vi "网分校准.vi"(8 "error in (no error)":errorcluster, 11 "network in":refnum<class "network.lvclass">) -> (0 "error out":errorcluster, 3 "network out":refnum<class "network.lvclass">)   [LabVIEW 2015, in "network.lvclass"]
uses:
  network.lvclass
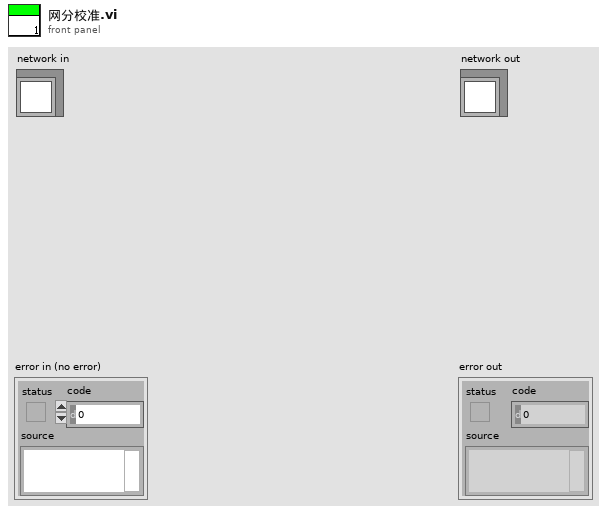
[diagram p1: front panel]
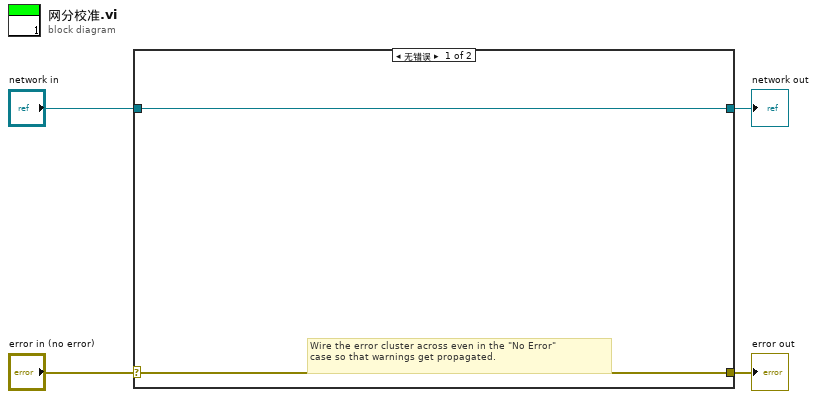
[diagram p0: block diagram]
diagram:
  n1 = case shown="无错误" "error in (no error)" {
    selector: "error in (no error)" -> [w5 w8]
    tunnel: [w5 w8] -> w3
    tunnel: [w6 w7] -> w1
    tunnel: "network in" -> [w6 w7]
    frame No Error {
      # "Wire the error cluster across even in the \"No Error\"\ncase so that warnings get propagated."
    }
    frame Error {
    }
  }
  "error out" <- w3
  "network out" <- w1
